vi "SeperateControlIndicatorRefs.vi"(8 "error in (no error)":errorcluster, 11 "Terminal references":refnum<vi>[](array[refnum])) -> (0 "error out":errorcluster, 2 "Indicator references":refnum<vi>[](array[refnum]), 3 "Control references":refnum<vi>[](array[refnum]))   [LabVIEW 2017, in "ErrorStructureDrawer.lvlib"]
doc: "Takes an array of control terminal references and seperates it into two new arrays: one for controls, and one for indicators."
uses:
  ErrorStructureDrawer.lvlib
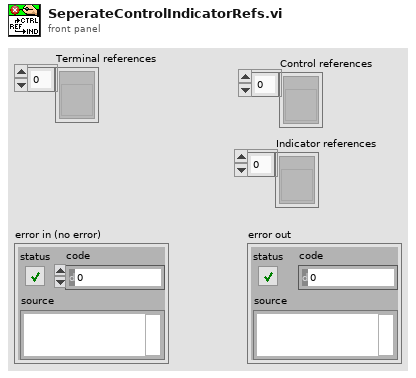
[diagram p1: front panel]
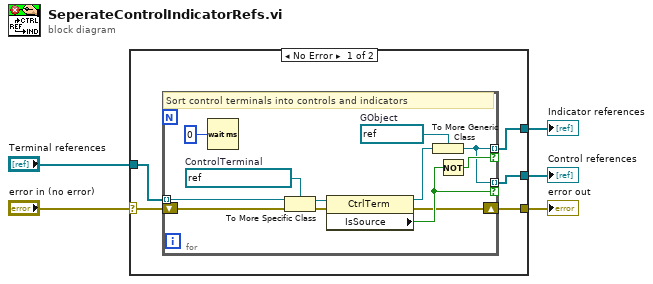
[diagram p0: block diagram]
diagram:
  n1 = case shown="No Error" "error in (no error)" {
    selector: "error in (no error)" -> [w6 w23]
    tunnel: [w10 w23] -> w5
    tunnel: "Terminal references" -> [w9 _]
    tunnel: [w8 _] -> w3
    tunnel: [w7 _] -> w2
    frame No Error {
      n2 = for {
        tunnel: w9 -> [w22] mode=indexing
        tunnel: [w16] -> w7 mode=indexing if=w18
        tunnel: [w16] -> w8 mode=indexing if=w19
        shift-right: [w11] -> w10
        shift-left: w6 -> [w12]
        w15 = refnum<vi> refnum  # GObject
        w21 = refnum<vi> refnum  # ControlTerminal
        # "Sort control terminals into controls and indicators"
        n3 = Wait (ms)(milliseconds to wait=u32 0) -> ()  [unwired: 1 out]
        n4 = To More Specific Class(target class=w21, reference=w22, error in=w12) -> (specific class reference=w20:refnum<vi>, error out=w13:errorcluster)
        n5 = property class="CtrlTerm"(reference=w20, error in=w13) -> (reference out=w17:refnum<vi>, error out=w11:errorcluster, "IsSource"=w18:bool)
        n6 = To More Generic Class(target class=w15, reference=w17) -> (generic class reference=w16:refnum<vi>)
        n7 = Not(x=w18) -> (.not. x?=w19:bool)
      }
    }
    frame Error {
    }
  }
  "error out" <- w5
  "Indicator references" <- w3
  "Control references" <- w2
